vi "Test DRAM FIFO.vi"() -> ()   [LabVIEW 2011]
uses:
  <instrlib>/FlexRIO/Libraries/Memory/FPGA/Interface/Timeslot Arbiter Configuration.ctl
  <instrlib>/RF-RIO/FIFO/FIFO/FPGA/Public/FIFO State.ctl
  <vilib>/Platform/TimedLoop/XDataNode/timing_clust.ctl
  <vilib>/Platform/TimedLoop/XDataNode/nitl_modes.ctl
  <vilib>/Platform/TimedLoop/XDataNode/wakeup.ctl
  <vilib>/Platform/TimedLoop/XDataNode/XDataNode.xnode
  <instrlib>/RF-RIO/FIFO/FIFO/FPGA/FIFO.lvlib
  <vilib>/Platform/TimedLoop/XDataNode/XDNodeRunTimeDep.lvlib
  <instrlib>/FlexRIO/Libraries/Memory/FPGA/Memory.lvlib
panel:
  out "Throughput (Bytes/sec)":u32
  out "bank0.data":T1
  out "Bank1.data":T1
  out "state":T2
  out "Bank1. Failed FIFO Data":u64
  out "Bank0.Failed FIFO Data":u64
  out "Failed Expected Data":u64
  out "Pass?":bool
  in  "arbiter configuration":T3={"write grant time (clocks)"=100, "read grant time (clocks)"=100}
  out "Check.Points Done":u32
  out "Gen. Points Done":u32
  in  "fifo depth":u8(ring)=8 items=["4"=2, "8"=3, "16"=4, "32"=5, "64"=6, "128"=7, "256"=8, "512"=9, "1024"=10, "2048"=11, "4096"=12, "8192"=13, "16384"=14, "32768"=15, "65536"=16, "131072"=17, "262144"=18, "524288"=19, "1048576"=20, "2097152"=21, "4194304"=22, "8388608"=23, "16777216"=24, "33554432"=25, "67108864"=26, "134217728"=27, "268435456"=28, "536870912"=29, "1073741824"=30, "2147483648"=31, "4294967296"=32]
  out "Generation Done?":bool
  in  "Points to Generate":u32
  out "Pattern Match Ever Fail?":bool
  out "Last Address Failed":u32
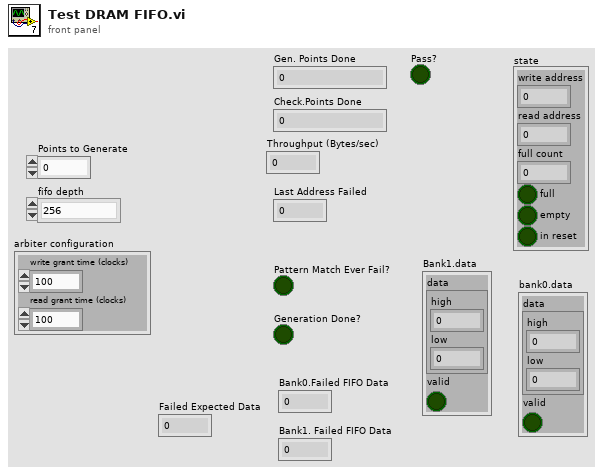
[diagram p1: front panel]
types:
  T1 = cluster{"data":cluster{"high":u64, "low":u64}, "valid":bool}
  T2 = typedef "FIFO.lvlib/FIFO State.ctl" = cluster{"write address":u32, "read address":u32, "full count":u32, "full":bool, "empty":bool, "in reset":bool}
  T3 = typedef "Memory.lvlib/Timeslot Arbiter Configuration.ctl" = cluster{"write grant time (clocks)":u16, "read grant time (clocks)":u16}
  T4 = typedef "XDNodeRunTimeDep.lvlib/timing_clust.ctl" = cluster{"Expected End [f-1]":u64, "Actual End [f-1]":u64, "Finished Late? [f-1]":bool, "Expected End [i-1]":u64, "Actual End [i-1]":u64, "Finished Late? [i-1]":bool, "Expected Start [i]":u64, "Actual Start [i]":u64, "Expected Start [f]":u64, "Actual Start [f]":u64, "Source Name":string, "Structure Name":string, "Period":i64, "Deadline":i64, "Offset":i64, "Start":i64, "Priority":i32, "Timeout":i32, "Mode":T5, "Wakeup Reason":T6, "Error":errorcluster, "Source Type":string, "Secondary Source Type":string, "Global End Time":u64, "Global Start Time":u64, "Frame Duration":u64, "Iteration Duration":u64, "Assigned CPU":i32, "I/O Scan Engine Mode":u32}
  T5 = typedef "XDNodeRunTimeDep.lvlib/nitl_modes.ctl" = enum32{"No Change", "Process missed periods, maintain original phase", "Discard missed periods, maintain original phase", "Process missed periods, ignore original phase", "Discard missed periods, ignore original phase"}
  T6 = typedef "XDNodeRunTimeDep.lvlib/wakeup.ctl" = enum32{"Normal", "Aborted", "Asynchronous wakeup", "Timing source error", "Timed loop error", "Timeout"}
  T7 = cluster{"fifo1 memory":refnum<k21>, "fifo2 memory":refnum<k21>}
  T8 = typedef "Data Type (256).ctl" = cluster{"Bank0. High":u64, "Bank0. Low":u64, "Bank1. High":u64, "Bank1. Low":u64}
  T9 = typedef "FIFO.lvlib/niRFRIO Memory 1.0.0 FPGA.lvlib/Retrieve Data (128-Bit).ctl" = cluster{"data":T10, "valid":bool}
  T10 = typedef "FIFO.lvlib/niRFRIO Memory 1.0.0 FPGA.lvlib/U128.ctl" = cluster{"high":u64, "low":u64}
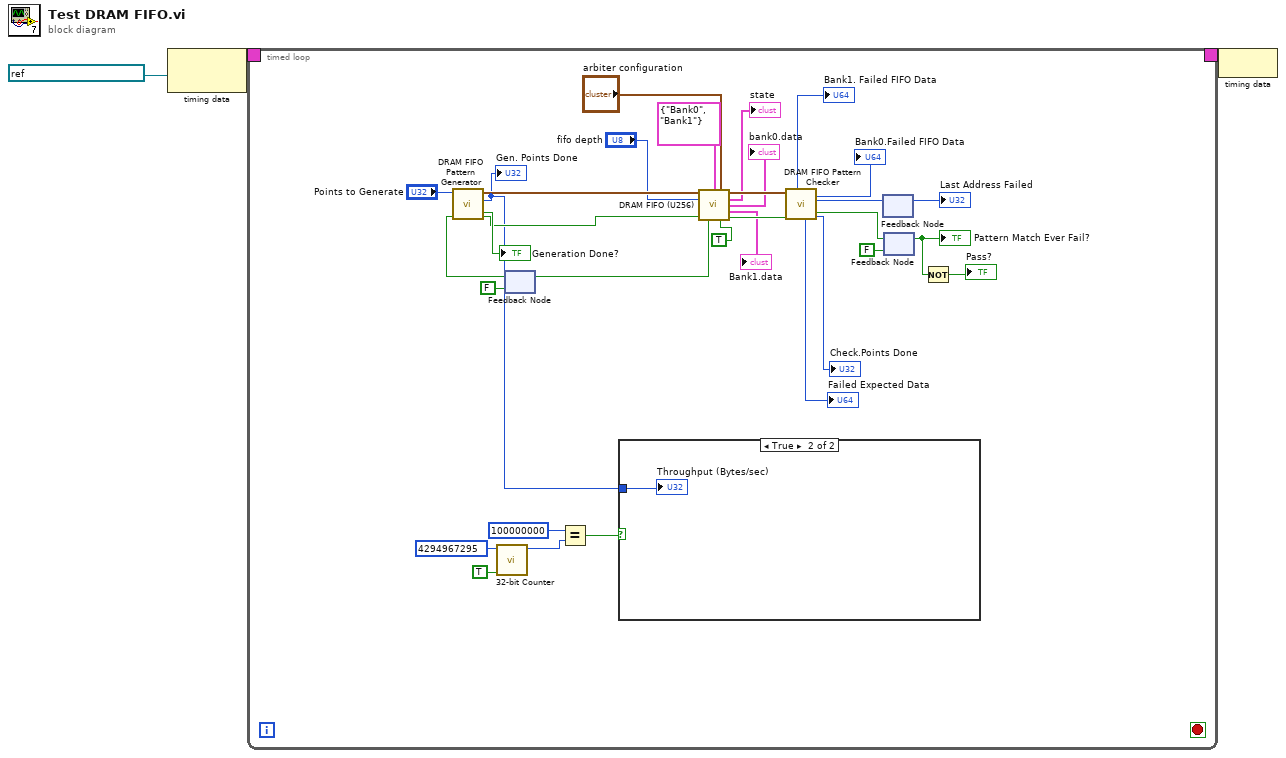
[diagram p0: block diagram]
diagram:
  n1 = node-c288(refnum<k21> "40 MHz Onboard Clock" ("Source Name")) -> (w3:T4)
  n2 = timed-loop {
    timing: w3 -> [_]
    timing-out: [_] -> w2
    stop <- _ stop-if-true
    n3 = call <userlib>:"32-bit Counter.vi"("INC?"=TRUE, "rollover"=u32 4294967295) -> ("count"=w10:u32)  [unwired: 9 in]
    n4 = feedback #1(FALSE ("Ready for Input")) -> (w33:bool)
    n5 = call <userlib>:"DRAM FIFO Pattern Generator.vi"("Generate Point"=w33, "Points to Generate"="Points to Generate") -> ("Output Valid"=w23:bool, "Generation Done?"=→"Generation Done?":bool, "Points Done"=w6:u32, "Output Data"=w34:T8)  [unwired: 6 in]
    "Gen. Points Done" <- w6
    n6 = Equal?(x=u32 100000000, y=w10) -> (x = y?=w11:bool)
    n7 = case shown="True" w11 {
      tunnel: w6 -> [_ w36]
      frame False {
      }
      frame True {
        "Throughput (Bytes/sec)" <- w36
      }
    }
    n8 = call <userlib>:"DRAM FIFO (U256).vi"("Input Data"=w34, "Memory"=T7 {"fifo1 memory"="Bank0", "fifo2 memory"="Bank1"}, "arbiter configuration"="arbiter configuration", "fifo depth"="fifo depth", "input valid"=w23, "ready for output"=TRUE) -> ("Output Data"=w21:T8, "state"=→"state":T2, "bank0.data"=→"bank0.data":T9, "Bank1.data"=→"Bank1.data":T9, "Ready for Input"=w5:bool, "Output Valid"=w20:bool)  [unwired: 4 in]
    n9 = feedback-in #1(w5) -> ()
    n10 = call <userlib>:"DRAM FIFO Pattern Checker.vi"("Input Valid"=w20, "Input Data"=w21) -> ("Points Done"=→"Check.Points Done":u32, "Pattern Match Ever Fail?"=w30:bool, "Last Address Failed"=w32:u32, "Expected Data"=→"Failed Expected Data":u64, "Bank0.Failed FIFO Data"=→"Bank0.Failed FIFO Data":u64, "Bank1. Failed FIFO Data"=→"Bank1. Failed FIFO Data":u64)  [unwired: 3 in, 1 out]
    n11 = feedback #2() -> (→"Last Address Failed":u32)  [unwired: 1 in]
    n12 = feedback-in #2(w32) -> ()
    n13 = feedback #3(FALSE ("Pattern Match Ever Fail?")) -> (w19:bool)
    "Pattern Match Ever Fail?" <- w19
    n14 = feedback-in #3(w30) -> ()
    n15 = Not(x=w19) -> (.not. x?=→"Pass?":bool)
  }
  n16 = node-c288(w2) -> ()
